vi "EEPROM Bulk Write test.vi"() -> ()   [LabVIEW 2010, in "lib1299.lvlib"]
uses:
  lib1299.lvlib
  <vilib>/Utility/config.llb/NI_LVConfig.lvlib
  <vilib>/Utility/config.llb/Read Key (String).vi
  <vilib>/Utility/config.llb/Write Key (String).vi
panel:
  in  "Write":bool
  out "Value that was written to the EEPROM data file":string
  in  "EEPROM Bulk Write Data":string[](array[string])=["ADS1278EVM", "12345-A", "12345-B", "12345-C", "12345-D"]
  out "Connected":bool=TRUE
  in  "Estyx device name":string
  in  "Firmware file":path
  out "Status box":string="Exiting"
  # "Device Name"
  # "PWB EDGE number and rev"
  # "PCA EDGE number and rev"
  # "BOM EDGE number and rev"
  # "Build Date"
  # "Device Name"
  # "PWB EDGE number and rev"
  # "PCA EDGE number and rev"
  # "BOM EDGE number and rev"
  # "Build Date"
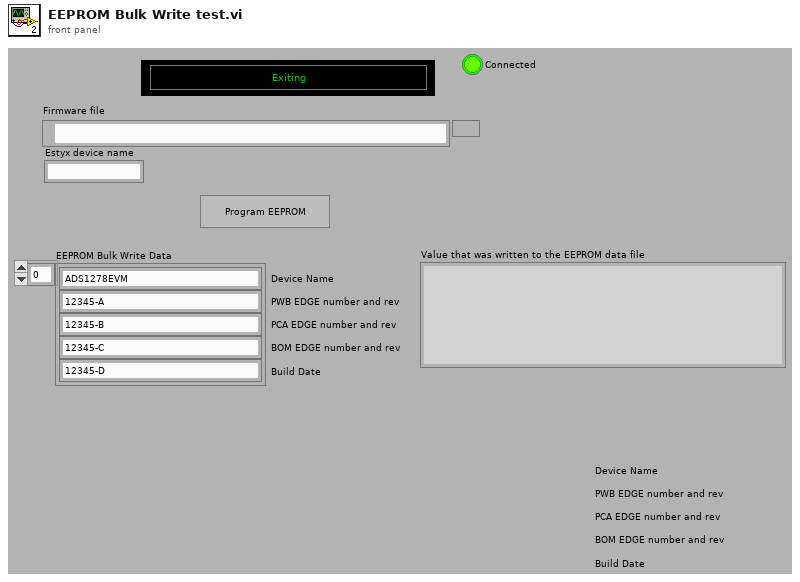
[diagram p1: front panel]
types:
  T1 = typedef "lib1299.lvlib/Tester states.ctl" = enum16{"Initialize", "File Check", "File New", "Load Firmware", "Save Firmware", "Operation", "Write Init", "Write Main", "Write Finish", "Read", "Wait", "Exit"}
  T2 = enum32{"invalid app kind", "Development System", "Run Time System", "Student Edition", "Embedded LabVIEW", "Evaluation", "Custom"}
  T3 = typedef "lib1299.lvlib/EEPROM Tester Info.ctl" = cluster{"client ptr":u32, "connection ptr":u32, "Firmware file":path, "Write VI Reference":refnum<vi>, "Estyx device name":string}
  T4 = typedef "NI_LVConfig.lvlib/Config Data RefNum.ctl" = refnum<k1>
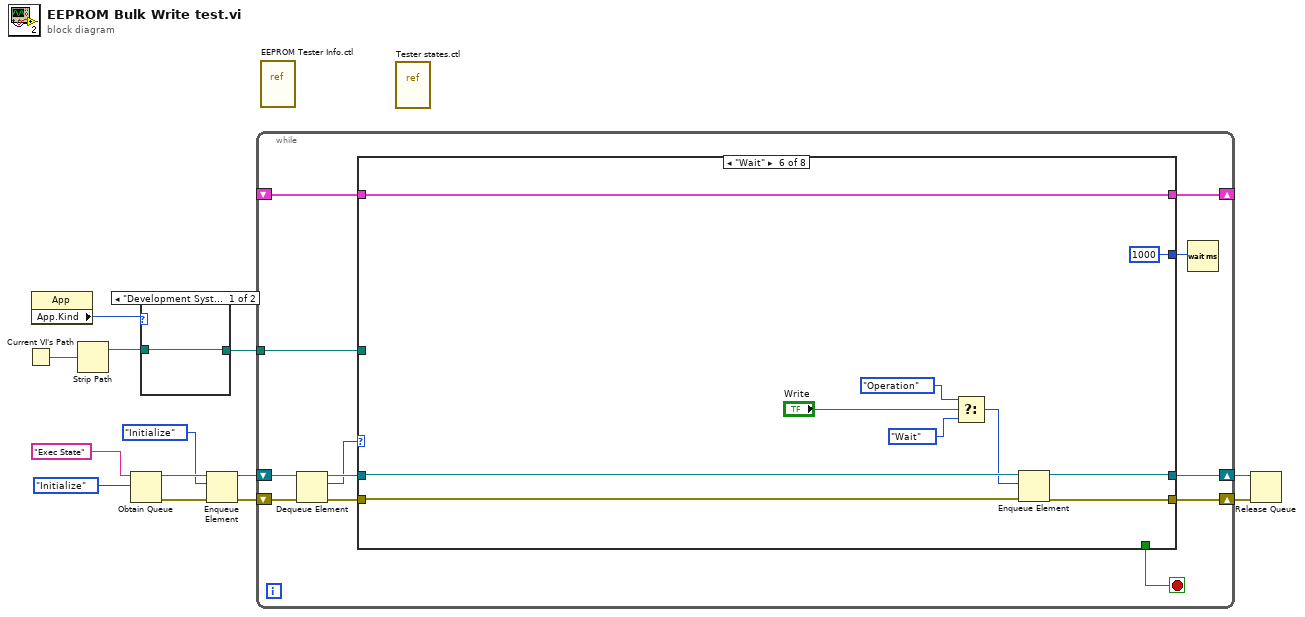
[diagram p0: block diagram]
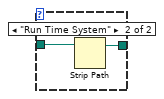
[diagram p2: hidden frame]
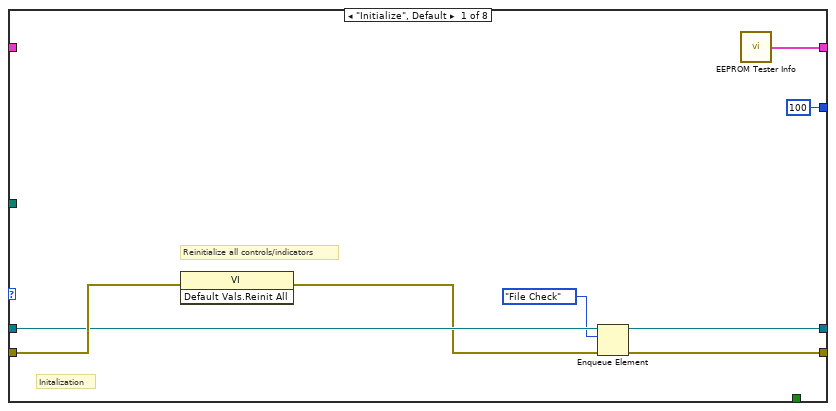
[diagram p3: hidden frame]
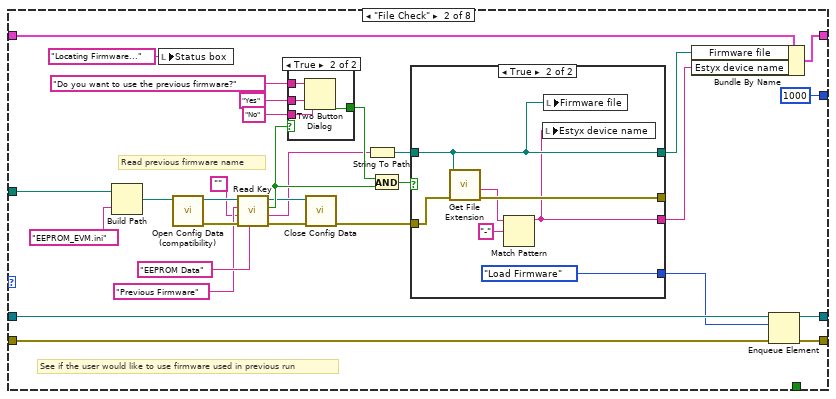
[diagram p4: hidden frame]
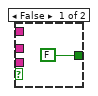
[diagram p5: hidden frame]
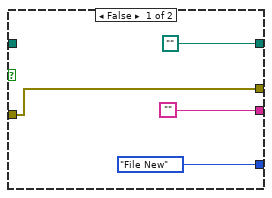
[diagram p6: hidden frame]
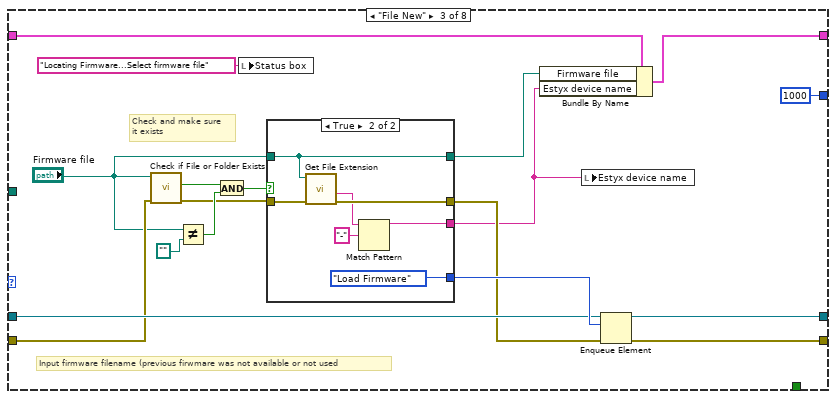
[diagram p7: hidden frame]
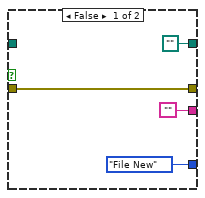
[diagram p8: hidden frame]
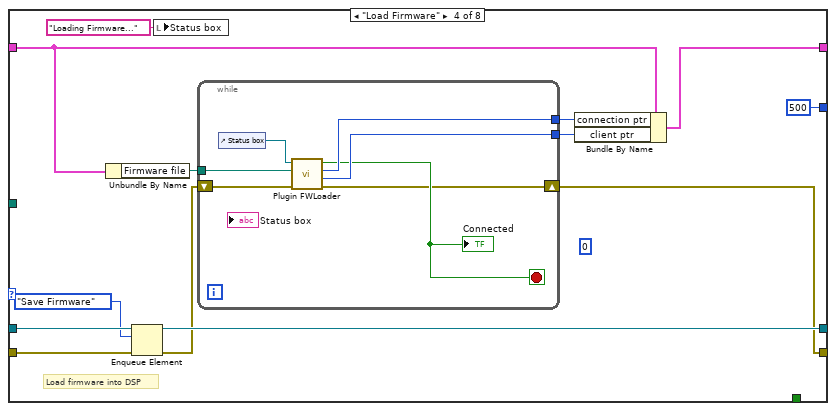
[diagram p9: hidden frame]
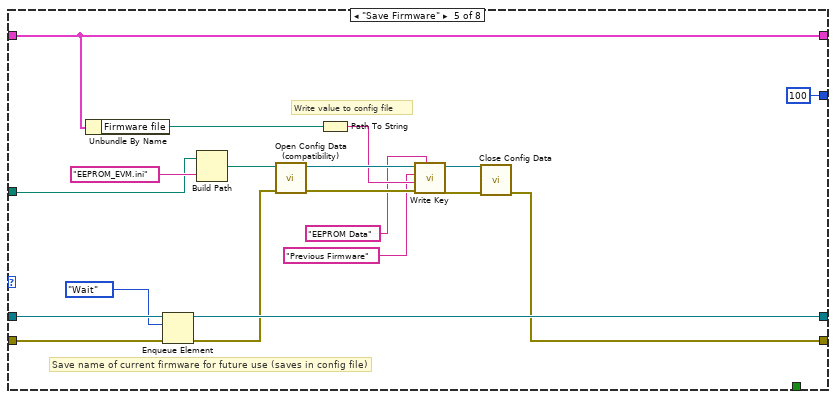
[diagram p10: hidden frame]
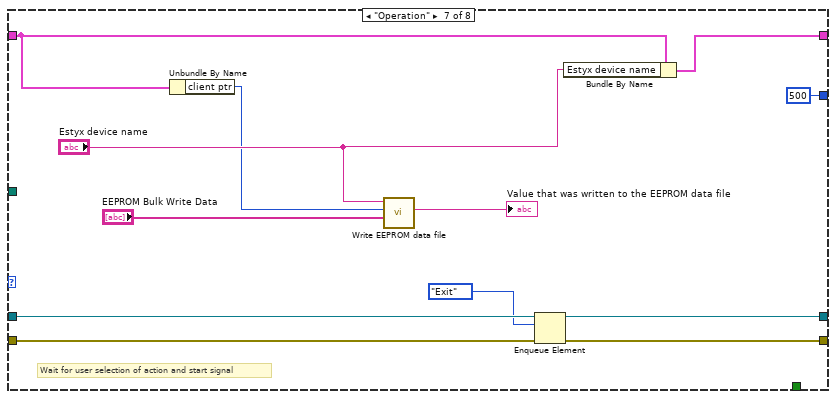
[diagram p11: hidden frame]
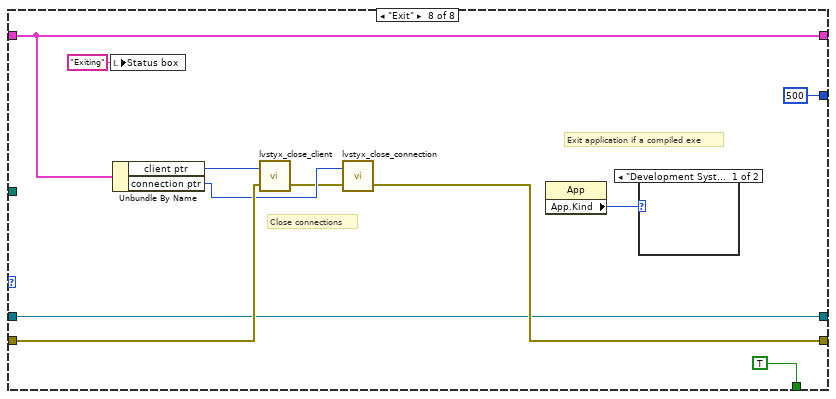
[diagram p12: hidden frame]
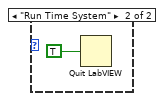
[diagram p13: hidden frame]
diagram:
  n1 = Current VI's Path() -> (path=w5:path)
  n2 = property class="App"() -> ("App.Kind"=w3:T2)  [unwired: 2 in, 2 out]
  n3 = Strip Path(path=w5) -> (stripped path=w6:path)  [unwired: 1 out]
  n4 = Obtain Queue(name (unnamed)="Exec State", element data type=Tester_states."Initialize" ("E2 test state")) -> (queue out=w10:refnum<queue>, error out=w13:errorcluster)  [unwired: 3 in, 1 out]
  n5 = case shown="\"Development System\", Default" w3 {
    tunnel: w6 -> [w14 w16]
    tunnel: [w14 w15] -> w4
    frame "Development System", Default {
    }
    frame "Run Time System" {
      n6 = Strip Path(path=w16) -> (stripped path=w15:path)  [unwired: 1 out]
    }
  }
  n7 = Enqueue Element(queue=w10, element=Tester_states."Initialize" ("E2 test state"), error in (no error)=w13) -> (queue out=w9:refnum<queue>, error out=w12:errorcluster)  [unwired: 1 in, 1 out]
  n8 = while {
    shift-right: [w19] -> w7
    shift-left: w12 -> [w28]
    shift-right: [w24] -> _
    shift-left: _ -> [w23]
    shift-right: [w20] -> w8
    shift-left: w9 -> [w27]
    tunnel: w4 -> [w18]
    stop <- w22 stop-if-true
    n9 = Dequeue Element(queue=w27, error in (no error)=w28) -> (queue out=w26:refnum<queue>, element=w21:T1, error out=w25:errorcluster)  [unwired: 1 in, 1 out]
    n10 = case shown="\"Wait\"" w21 {
      tunnel: w26 -> [w35 w65 w98 w124 w150 w157 w171 w179]
      tunnel: w25 -> [w36 w62 w89 w123 w149 w158 w172 w180]
      tunnel: [w33 w66 w99 w112 w134 w159 w165 w182] -> w19
      tunnel: [w32 w63 w91 w118 w148 w160 w170 w179] -> w20
      tunnel: [w29 w64 w97 w120 w137 w151 w169 w183] -> w24
      tunnel: w23 -> [_ w37 w86 w121 w137 w151 w167 w183]
      tunnel: [_ _ _ _ _ _ _ TRUE] -> w22
      tunnel: w18 -> [_ w56 _ _ w138 _ _ _]
      tunnel: [u32 100 ("milliseconds to wait") u32 1000 ("milliseconds to wait") u32 1000 ("milliseconds to wait") u32 500 ("milliseconds to wait") u32 100 ("milliseconds to wait") u32 1000 ("milliseconds to wait") u32 500 ("milliseconds to wait") u32 500 ("milliseconds to wait")] -> w17
      frame "Initialize", Default {
        # "Initalization"
        # "Reinitialize all controls/indicators"
        n11 = invoke class="VI" method="Default Vals.Reinit All"(error in=w36) -> (error out=w34:errorcluster)  [unwired: 2 in, 2 out]
        n12 = Enqueue Element(queue=w35, element=Tester_states."File Check" ("E2 test state"), error in (no error)=w34) -> (queue out=w32:refnum<queue>, error out=w33:errorcluster)  [unwired: 1 in, 1 out]
        n13 = call "EEPROM Tester Info.vi"() -> ("EEPROM Tester Info"=w29:T3)  [unwired: 1 in]
      }
      frame "File Check" {
        # "Read previous firmware name"
        # "See if the user would like to use firmware used in previous run"
        n14 = Build Path(base path=w56, name or relative path="EEPROM_EVM.ini") -> (appended path=w54:path)
        n15 = local write "Status box"("Locating Firmware..." ("Status box")) -> ()
        n16 = call <vilib>:"Open Config Data (compatibility).vi"("configuration file path"=w54) -> ("error out"=w59:errorcluster, "refnum"=w60:T4)  [unwired: 8 in, 1 out]
        n17 = call-poly <vilib>:"Read Key.vi"("section"="EEPROM Data", "error in (no error)"=w59, "default value"="", "key"="Previous Firmware" ("section"), "refnum"=w60) -> ("error out"=w45:errorcluster, "value"=w42:string, "found?"=w46:bool, "refnum out"=w43:T4)  [unwired: 3 in]
        n18 = case shown="True" w46 {
          tunnel: "Do you want to use the previous firmware?" ("message") -> [_ w71]
          tunnel: "Yes" ("T button name (\"OK\")") -> [_ w70]
          tunnel: "No" ("F button name (\"Cancel\")") -> [_ w69]
          tunnel: [FALSE ("T button?") w68] -> w47
          frame False {
          }
          frame True {
            n19 = Two Button Dialog(message=w71, 1:w69, 2:w70) -> (T button?=w68:bool)
          }
        }
        n20 = call <vilib>:"Close Config Data.vi"("error in (no error)"=w45, "refnum"=w43) -> ("error out"=w44:errorcluster)  [unwired: 8 in, 1 out]
        n21 = String To Path(string=w42) -> (path=w41:path)
        n22 = And(x=w47, y=w46) -> (x .and. y?=w48:bool)
        n23 = case shown="True" w48 {
          tunnel: [Tester_states."File New" ("E2 test state") Tester_states."Load Firmware" ("E2 test state")] -> w53
          tunnel: [path "" w79] -> w52
          tunnel: w41 -> [_ w79]
          tunnel: [w73 w82] -> _
          tunnel: ["" w77] -> w40
          tunnel: w44 -> [w73 w80]
          frame False {
          }
          frame True {
            n24 = call <vilib>:"Get File Extension.vi"("error in (no error)"=w80, "file"=w79) -> ("error out"=w82:errorcluster, "filename without extension"=w78:string)  [unwired: 6 in, 2 out]
            n25 = Match Pattern(string=w78, regular expression="-") -> (before substring=w77:string)  [unwired: 1 in, 3 out]
            n26 = local write "Estyx device name"(w77) -> ()
            n27 = local write "Firmware file"(w79) -> ()
          }
        }
        n28 = Bundle By Name(cluster=w37, "Firmware file"=w52, "Estyx device name"=w40) -> (w64:T3)
        n29 = Enqueue Element(queue=w65, element=w53, error in (no error)=w62) -> (queue out=w63:refnum<queue>, error out=w66:errorcluster)  [unwired: 1 in, 1 out]
      }
      frame "File New" {
        # "Check and make sure\nit exists"
        # "Input firmware filename (previous firwmare was not available or not used"
        n30 = call <vilib>:"Check if File or Folder Exists.vi"("error in (no error)"=w89, "path"="Firmware file") -> ("error out"=w90:errorcluster, "file or folder exists?"=w94:bool)  [unwired: 7 in, 1 out]
        n31 = Not Equal?(x="Firmware file", y=path "") -> (x != y?=w93:bool)
        n32 = And(x=w94, y=w93) -> (x .and. y?=w95:bool)
        n33 = local write "Status box"("Locating Firmware...Select firmware file" ("Status box")) -> ()
        n34 = case shown="True" w95 {
          tunnel: [Tester_states."File New" ("E2 test state") Tester_states."Load Firmware" ("E2 test state")] -> w100
          tunnel: [path "" w111] -> w96
          tunnel: "Firmware file" -> [_ w111]
          tunnel: w90 -> [w103 w110]
          tunnel: [w103 w109] -> w88
          tunnel: ["" w107] -> w87
          frame False {
          }
          frame True {
            n35 = call <vilib>:"Get File Extension.vi"("error in (no error)"=w110, "file"=w111) -> ("error out"=w109:errorcluster, "filename without extension"=w108:string)  [unwired: 6 in, 2 out]
            n36 = Match Pattern(string=w108, regular expression="-") -> (before substring=w107:string)  [unwired: 1 in, 3 out]
          }
        }
        n37 = Bundle By Name(cluster=w86, "Firmware file"=w96, "Estyx device name"=w87) -> (w97:T3)
        n38 = local write "Estyx device name"(w87) -> ()
        n39 = Enqueue Element(queue=w98, element=w100, error in (no error)=w88) -> (queue out=w91:refnum<queue>, error out=w99:errorcluster)  [unwired: 1 in, 1 out]
      }
      frame "Load Firmware" {
        (unwired) u8 0 ("Disabled")
        # "Load firmware into DSP"
        n40 = Unbundle By Name(w121) -> ("Firmware file"=w122:path)
        n41 = Enqueue Element(queue=w124, element=Tester_states."Save Firmware" ("E2 test state"), error in (no error)=w123) -> (queue out=w118:refnum<queue>, error out=w113:errorcluster)  [unwired: 1 in, 1 out]
        n42 = local write "Status box"("Loading Firmware..." ("Status box")) -> ()
        n43 = while {
          tunnel: [w130] -> w119
          tunnel: w122 -> [w131]
          tunnel: [w129] -> w117
          shift-right: [w126] -> w112
          shift-left: w113 -> [w125]
          stop <- w128 stop-if-true
          n44 = control-ref of="Status box"() -> (w127:refnum<vi>)
          n45 = call "Plugin FWLoader.vi"("error in (no error)"=w125, "Firmware file"=w131, "Status reference"=w127) -> ("error out"=w126:errorcluster, "client ptr"=w129:i32, "connection ptr"=w130:i32, "Connected"=w128:bool)  [unwired: 1 in]
          "Connected" <- w128
        }
        n46 = Bundle By Name(cluster=w121, "connection ptr"=w119, "client ptr"=w117) -> (w120:T3)
      }
      frame "Save Firmware" {
        # "Write value to config file"
        # "Save name of current firmware for future use (saves in config file)"
        n47 = Unbundle By Name(w137) -> ("Firmware file"=w136:path)
        n48 = Enqueue Element(queue=w150, element=Tester_states."Wait" ("E2 test state"), error in (no error)=w149) -> (queue out=w148:refnum<queue>, error out=w135:errorcluster)  [unwired: 1 in, 1 out]
        n49 = Build Path(base path=w138, name or relative path="EEPROM_EVM.ini") -> (appended path=w143:path)
        n50 = call <vilib>:"Open Config Data (compatibility).vi"("error in (no error)"=w135, "configuration file path"=w143) -> ("error out"=w147:errorcluster, "refnum"=w146:T4)  [unwired: 7 in, 1 out]
        n51 = Path To String(path=w136) -> (string=w141:string)
        n52 = call-poly <vilib>:"Write Key.vi"("section"="EEPROM Data", "error in (no error)"=w147, "value"=w141, "key"="Previous Firmware" ("section"), "refnum"=w146) -> ("error out"=w144:errorcluster, "refnum out"=w145:T4)  [unwired: 4 in, 1 out]
        n53 = call <vilib>:"Close Config Data.vi"("error in (no error)"=w144, "refnum"=w145) -> ("error out"=w134:errorcluster)  [unwired: 8 in, 1 out]
      }
      frame "Wait" {
        n54 = Select(t=Tester_states."Operation", s="Write", f=Tester_states."Wait" ("E2 test state")) -> (s? t:f=w154:T1)
        n55 = Enqueue Element(queue=w157, element=w154, error in (no error)=w158) -> (queue out=w160:refnum<queue>, error out=w159:errorcluster)  [unwired: 1 in, 1 out]
      }
      frame "Operation" {
        # "Wait for user selection of action and start signal"
        n56 = Unbundle By Name(w167) -> ("client ptr"=w163:u32)
        n57 = call "Write EEPROM data file.vi"("EEPROM files to write"="EEPROM Bulk Write Data", "client ptr"=w163, "Estyx device name"="Estyx device name") -> ("To be written to the data file"=→"Value that was written to the EEPROM data file":string)  [unwired: 7 in, 1 out]
        n58 = Enqueue Element(queue=w171, element=Tester_states."Exit" ("E2 test state"), error in (no error)=w172) -> (queue out=w170:refnum<queue>, error out=w165:errorcluster)  [unwired: 1 in, 1 out]
        n59 = Bundle By Name(cluster=w167, "Estyx device name"="Estyx device name") -> (w169:T3)
      }
      frame "Exit" {
        # "Exit application if a compiled exe"
        # "Close connections"
        n60 = local write "Status box"("Exiting" ("Status box")) -> ()
        n61 = Unbundle By Name(w183) -> ("client ptr"=w177:u32, "connection ptr"=w176:u32)
        n62 = call "lvstyx_close_client.vi"("error in (no error)"=w180, "client ptr"=w177) -> ("error out"=w175:errorcluster)  [unwired: 1 in]
        n63 = call "lvstyx_close_connection.vi"("error in (no error)"=w175, "connection ptr"=w176) -> ("error out"=w182:errorcluster)  [unwired: 1 in]
        n64 = property class="App"() -> ("App.Kind"=w173:T2)  [unwired: 2 in, 2 out]
        n65 = case shown="\"Development System\", Default" w173 {
          frame "Development System", Default {
          }
          frame "Run Time System" {
            n66 = Quit LabVIEW(quit? (T)=TRUE) -> ()
          }
        }
      }
    }
    n67 = Wait (ms)(milliseconds to wait=w17) -> ()  [unwired: 1 out]
  }
  n68 = vi-ref "EEPROM Tester Info.ctl"() -> ()  [unwired: 1 out]
  n69 = vi-ref "Tester states.ctl"() -> ()  [unwired: 1 out]
  n70 = Release Queue(queue=w8, error in (no error)=w7) -> ()  [unwired: 1 in, 3 out]
